vi "Stop Serial Port.vi"(0 "FPGA Main Ref":refnum<k20>, 11 "Error IN":errorcluster) -> (15 "Error OUT":errorcluster)   [LabVIEW 2011]
uses:
  <vilib>/Utility/error.llb/Error Cluster From Error Code.vi
  <vilib>/rvi/errors/niLvFpgaAdjustHostInterfaceError.vi
  <vilib>/FPGAPlugInAG/sbRIO-9606/niLvFpga_Close_sbRIO-9606.vi
  <vilib>/rvi/interface/nirviReadWriteControl/nirviReadWriteControl.xnode
  FPGA Bitfiles/JAGM_FPGATarget_FPGAMain_A31A659D.lvbitx
  FPGA Source/FPGA Main.vi
  <vilib>/rvi/interface/nirviCloseFPGA/nirviCloseFPGA.xnode
  NiFpgaLv.dll
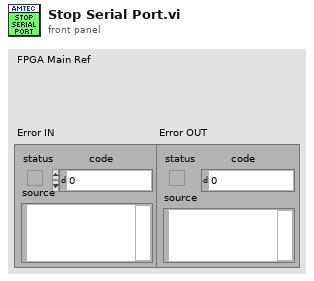
[diagram p1: front panel]
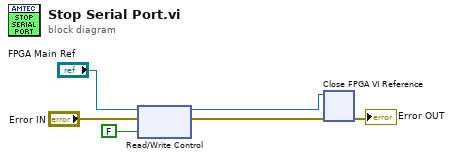
[diagram p0: block diagram]
diagram:
  n1 = xnode "Read/Write Control"("FPGA VI Reference In"="FPGA Main Ref", "error in"="Error IN", "Read"=FALSE ("stop")) -> ("FPGA VI Reference Out"=w1:refnum<k20>, "error out"=w5:errorcluster)
  n2 = xnode "Close FPGA VI Reference"("FPGA VI Reference In"=w1, "error in"=w5) -> ("error out"=→"Error OUT":errorcluster)
